vi "Compile Inline Execution Units.vi"(8 "error in":errorcluster, 10 "Inline Execution Units":T5[](array[typedef]) {"ReadWrite Channels" format="%.0x"; "Outgoing Channels" format="%.0x"; "Incoming Channels" format="%.0x"}, 11 "Device Ref in":T4=18446744073709551615 format="%.0x") -> (0 "error out":errorcluster, 2 "Compiled Inline Execution Units":T1[](array[typedef]) {"Outgoing Data References"."Data Reference" format="%.0x"; "Incoming Data References" format="%.0x"}, 3 "Device Ref out":T4=18446744073709551615 format="%.0x")   [LabVIEW 2020, in "AIM MIL-STD-1553 System Explorer.lvlib"]
uses:
  AIM MIL-STD-1553 System Explorer.lvlib
  Includes/AIM MIL-STD-1553 Engine.lvlibp/Engine/Interfaces/Controls/Execution Unit Information.ctl
  Includes/AIM MIL-STD-1553 Engine.lvlibp/Engine/Interfaces/Execution Unit/Execution Unit.lvclass
  Includes/AIM MIL-STD-1553 Engine.lvlibp/1abvi3w/vi.lib/NI VeriStand/Custom Device API/Custom Device Item Ref.ctl
  <vilib>/NI VeriStand/Custom Device API/Custom Device Item Ref.ctl
  Shared/Inline Execution Unit Compiled Information.ctl
  <vilib>/NI VeriStand/Custom Device API/Data Reference.ctl
  <vilib>/NI VeriStand/Custom Device API/Block Data Reference.ctl
  <vilib>/NI VeriStand/Custom Device API/Data Access Type.ctl
  <vilib>/NI VeriStand/Custom Device API/Custom Device API.lvlib
  Shared/AIM MIL-STD-1553 Shared.lvlib
  Includes/AIM MIL-STD-1553 Engine.lvlibp/Engine/Interfaces/Interfaces.lvlib
  Includes/AIM MIL-STD-1553 Engine.lvlibp/1abvi3w/vi.lib/NI VeriStand/Custom Device API/Custom Device API.lvlib
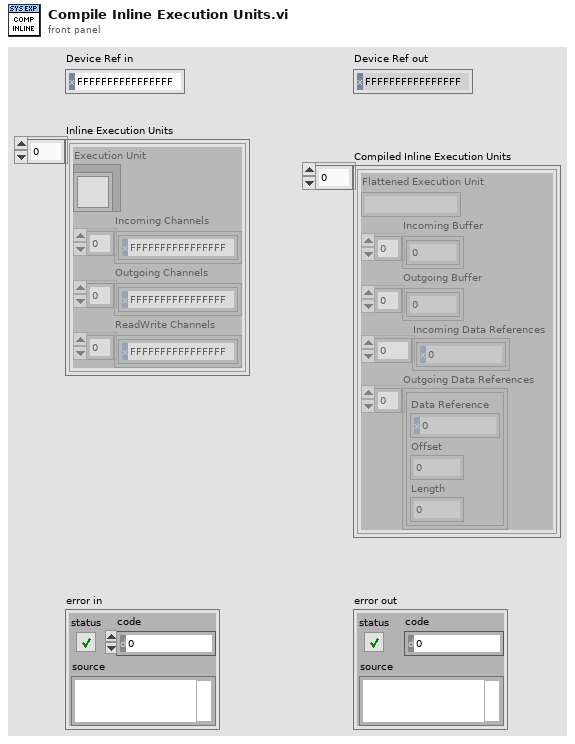
[diagram p1: front panel]
types:
  T1 = typedef "AIM MIL-STD-1553 Shared.lvlib/Inline Execution Unit Compiled Information.ctl" = cluster{"Flattened Execution Unit":string, "Incoming Buffer":dbl[], "Outgoing Buffer":dbl[], "Incoming Data References":T2[], "Outgoing Data References":T3[]}
  T2 = typedef "Custom Device API.lvlib/Data Reference.ctl" = i32
  T3 = typedef "Custom Device API.lvlib/Block Data Reference.ctl" = cluster{"Data Reference":T2, "Offset":u64, "Length":u64}
  T4 = typedef "Custom Device API.lvlib/Custom Device Item Ref.ctl" = u64
  T5 = typedef "AIM MIL-STD-1553 Engine.lvlibp/Interfaces.lvlib/Execution Unit Information.ctl" = cluster{"Execution Unit":refnum<class "Execution Unit.lvclass">, "Incoming Channels":T6[], "Outgoing Channels":T6[], "ReadWrite Channels":T6[]}
  T6 = typedef "AIM MIL-STD-1553 Engine.lvlibp/Custom Device API.lvlib/Custom Device Item Ref.ctl" = u64
  T7 = typedef "Custom Device API.lvlib/Data Access Type.ctl" = enum16{"Read", "Write"}
  T8 = typedef "Custom Device API.lvlib/Custom Device Channel.ctl" = cluster{"Type":T9, "Units":string, "Default Value":dbl, "Faultable":bool, "Scalable":bool}
  T9 = typedef "Custom Device API.lvlib/Custom Device Channel Type.ctl" = enum16{"Input", "Output"}
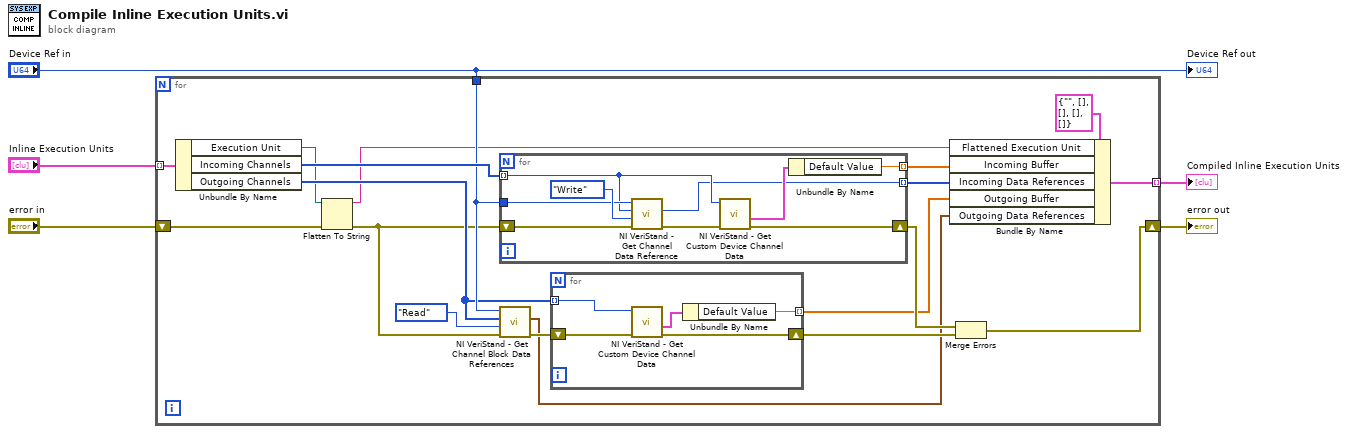
[diagram p0: block diagram]
diagram:
  n1 = for {
    tunnel: "Inline Execution Units" -> [w23] mode=indexing
    tunnel: "Device Ref in" -> [w22]
    tunnel: [w9] -> w1 mode=indexing
    shift-right: [w10] -> w2
    shift-left: "error in" -> [w15]
    n2 = Unbundle By Name(w23) -> ("Execution Unit"=w7:refnum<class "Execution Unit.lvclass">, "Incoming Channels"=w24:T6[], "Outgoing Channels"=w19:T6[])
    n3 = Flatten To String(anything=w7, error in (no error)=w15) -> (data string=w6:string, error out=w8:errorcluster)  [unwired: 2 in, 1 out]
    n4 = for {
      tunnel: w24 -> [w35] mode=indexing
      tunnel: w22 -> [w37]
      shift-right: [w32] -> w14
      shift-left: w8 -> [w33]
      tunnel: [w31] -> w17 mode=indexing
      tunnel: [w30] -> w16 mode=indexing
      n5 = call <vilib>:"NI VeriStand - Get Channel Data Reference.vi"("error in (no error)"=w33, "Access"=Data_Access_Type."Write", "Channel Ref in"=w35, "Device Ref in"=w37) -> ("error out"=w34:errorcluster, "Channel Data Reference"=w30:T2)  [unwired: 5 in, 1 out]
      n6 = call <vilib>:"NI VeriStand - Get Custom Device Channel Data.vi"("error in (no error)"=w34, "Channel Ref in"=w35) -> ("error out"=w32:errorcluster, "Channel"=w36:T8)  [unwired: 4 in, 4 out]
      n7 = Unbundle By Name(w36) -> ("Default Value"=w31:dbl)
    }
    n8 = call <vilib>:"NI VeriStand - Get Channel Block Data References.vi"("error in (no error)"=w8, "Access"=Data_Access_Type."Read", "Channel Refs"=w19, "Device Ref in"=w22) -> ("error out"=w20:errorcluster, "Block Data Refs"=w12:T3[])  [unwired: 4 in, 2 out]
    n9 = for {
      shift-right: [w28] -> w13
      shift-left: w20 -> [w29]
      tunnel: w19 -> [w27] mode=indexing
      tunnel: [w25] -> w11 mode=indexing
      n10 = call <vilib>:"NI VeriStand - Get Custom Device Channel Data.vi"("error in (no error)"=w29, "Channel Ref in"=w27) -> ("error out"=w28:errorcluster, "Channel"=w26:T8)  [unwired: 4 in, 4 out]
      n11 = Unbundle By Name(w26) -> ("Default Value"=w25:dbl)
    }
    n12 = Bundle By Name(cluster=T1 {"Flattened Execution Unit"="", "Incoming Buffer"=[], "Outgoing Buffer"=[], "Incoming Data References"=[], "Outgoing Data References"=[]} ("Execution Unit Compiled Information"), "Flattened Execution Unit"=w6, "Incoming Buffer"=w17, "Incoming Data References"=w16, "Outgoing Buffer"=w11, "Outgoing Data References"=w12) -> (w9:T1)
    n13 = Merge Errors(w14, w13) -> (w10:errorcluster)
  }
  "error out" <- w2
  "Compiled Inline Execution Units" <- w1
  "Device Ref out" <- "Device Ref in"
